vi "Push Buffer to Sink.vi"(8 "error in (no error)":errorcluster, 10 "Strings to Log":string[](array[string]), 11 "Buffered Log Sink in":refnum<class "Buffered String Log Sink.lvclass">) -> (0 "error out":errorcluster, 3 "Buffered Log Sink out":refnum<class "Buffered String Log Sink.lvclass">)   [LabVIEW 2020, in "MVA Framework.lvlib" / "Buffered String Log Sink.lvclass"]
uses:
  Buffered String Log Sink.lvclass
  Buffered String Log Sink.lvclass/Buffered String Log Sink.ctl
  String Log Sink/String Log Sink.lvclass
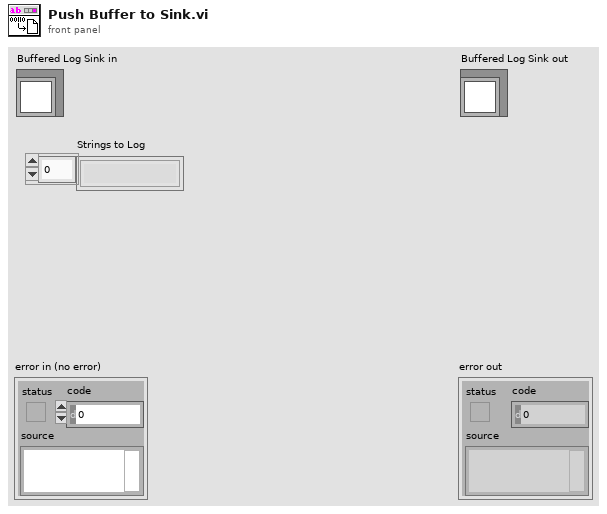
[diagram p1: front panel]
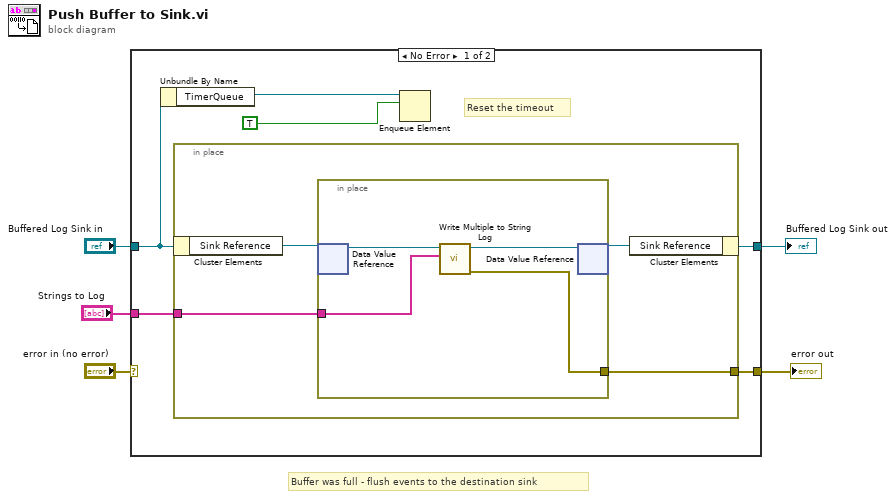
[diagram p0: block diagram]
diagram:
  # "Buffer was full - flush events to the destination sink"
  n1 = case shown="No Error" "error in (no error)" {
    selector: "error in (no error)" -> [_ w20]
    tunnel: "Buffered Log Sink in" -> [w9 w21]
    tunnel: [w11 w21] -> w4
    tunnel: [w10 w20] -> w2
    tunnel: "Strings to Log" -> [w6 _]
    frame No Error {
      # "Reset the timeout"
      n2 = Unbundle By Name(w9) -> ("TimerQueue"=w8:refnum<queue>)
      n3 = in-place {
        in-place-border: [w15] -> w10
        in-place-border: w6 -> [w12]
        n4 = in-place-cluster #1(w9) -> ("Sink Reference"=w14:refnum<data-value>)
        n5 = in-place {
          in-place-border: [w17] -> w15
          in-place-border: w12 -> [w16]
          n6 = in-place-dvr #2(w14) -> (w19:refnum<class "String Log Sink.lvclass">)  [unwired: 1 out]
          n7 = call-dynamic "Write Multiple to String Log.vi"("Strings to Log"=w16, "String Log Sink in"=w19) -> ("error out"=w17:errorcluster, "String Log Sink out"=w18:refnum<class "String Log Sink.lvclass">)  [unwired: 8 in]
          n8 = in-place-dvr #2(w18) -> (w13:refnum<data-value>)  [unwired: 1 out]
        }
        n9 = in-place-cluster #1("Sink Reference"=w13) -> (w11:refnum<class "Buffered String Log Sink.lvclass">)
      }
      n10 = Enqueue Element(queue=w8, element=TRUE) -> ()  [unwired: 2 in, 3 out]
    }
    frame Error {
    }
  }
  "error out" <- w2
  "Buffered Log Sink out" <- w4
